vi "Loop.vi"(9 "Error Queue":refnum<queue>, 10 "Helper Loop Queue":refnum<queue>, 11 "Helper Loop in":refnum<class "jettl Event Actor.lvclass">) -> ()   [LabVIEW 2021, in "jettl Event Actor.lvclass"]
uses:
  jettl Event Actor.lvclass
  Event Actor/Event Actor.lvclass
  jettl Event Actor.lvclass/jettl Event Actor.ctl
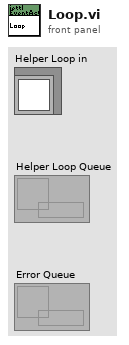
[diagram p1: front panel]
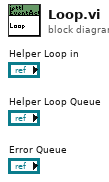
[diagram p0: block diagram]
diagram:
